vi "Protobuf decoder.vi"(8 "error in (no error)":errorcluster, 10 "String":string) -> (0 "error out":errorcluster, 2 "Cluster":T1)   [LabVIEW 2020]
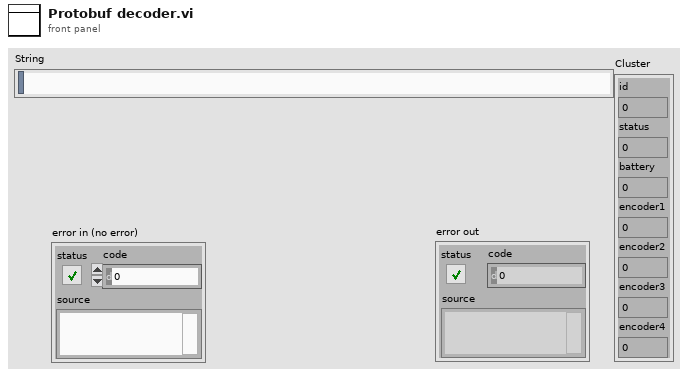
[diagram p1: front panel]
types:
  T1 = cluster{"id":u32, "status":u32, "battery":sgl, "encoder1":sgl, "encoder2":sgl, "encoder3":sgl, "encoder4":sgl}
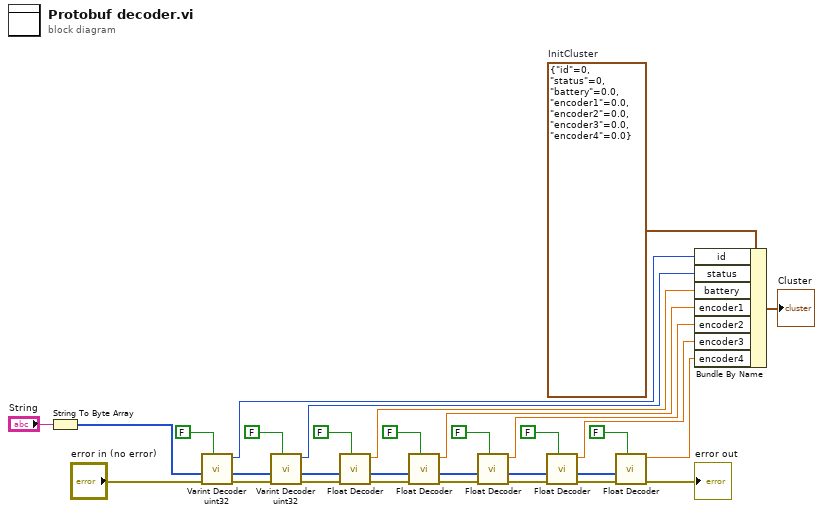
[diagram p0: block diagram]
diagram:
  w31 = T1 {"id"=0, "status"=0, "battery"=0.0, "encoder1"=0.0, "encoder2"=0.0, "encoder3"=0.0, "encoder4"=0.0}  # InitCluster
  n1 = String To Byte Array(string="String") -> (unsigned byte array=w26:u8[])
  n2 = call "Varint Decoder uint32.vi"("Optional"=FALSE, "error in (no error)"="error in (no error)", "Array"=w26) -> ("error out"=w22:errorcluster, "array w/ subset deleted"=w23:u8[], "Varint"=w28:u32)  [unwired: 5 in, 1 out]
  n3 = call "Varint Decoder uint32.vi"("Optional"=FALSE, "error in (no error)"=w22, "Array"=w23) -> ("error out"=w18:errorcluster, "array w/ subset deleted"=w19:u8[], "Varint"=w24:u32)  [unwired: 5 in, 1 out]
  n4 = call "Float Decoder.vi"("Optional"=FALSE, "error in (no error)"=w18, "Array"=w19) -> ("error out"=w14:errorcluster, "array w/ subset deleted"=w15:u8[], "Float"=w20:sgl)  [unwired: 5 in, 1 out]
  n5 = call "Float Decoder.vi"("Optional"=FALSE, "error in (no error)"=w14, "Array"=w15) -> ("error out"=w10:errorcluster, "array w/ subset deleted"=w11:u8[], "Float"=w16:sgl)  [unwired: 5 in, 1 out]
  n6 = call "Float Decoder.vi"("Optional"=FALSE, "error in (no error)"=w10, "Array"=w11) -> ("error out"=w6:errorcluster, "array w/ subset deleted"=w7:u8[], "Float"=w12:sgl)  [unwired: 5 in, 1 out]
  n7 = call "Float Decoder.vi"("Optional"=FALSE, "error in (no error)"=w6, "Array"=w7) -> ("error out"=w2:errorcluster, "array w/ subset deleted"=w3:u8[], "Float"=w8:sgl)  [unwired: 5 in, 1 out]
  n8 = call "Float Decoder.vi"("Optional"=FALSE, "error in (no error)"=w2, "Array"=w3) -> ("error out"=→"error out":errorcluster, "Float"=w4:sgl)  [unwired: 5 in, 2 out]
  n9 = Bundle By Name(cluster=w31, "id"=w28, "status"=w24, "battery"=w20, "encoder1"=w16, "encoder2"=w12, "encoder3"=w8, "encoder4"=w4) -> (→"Cluster":T1)
